vi "Calculate psrr.vi"(8 "error in (no error)":errorcluster, 11 "Time signal(s) in":waveform(dbl)[](array[waveform])) -> (0 "error out":errorcluster, 2 "PSRR":dbl)   [LabVIEW 2021]
uses:
  <vilib>/measure/madcrms.llb/Basic Averaged DC-RMS for N Chan.vi
  <vilib>/measure/NI_MAPro.lvlib
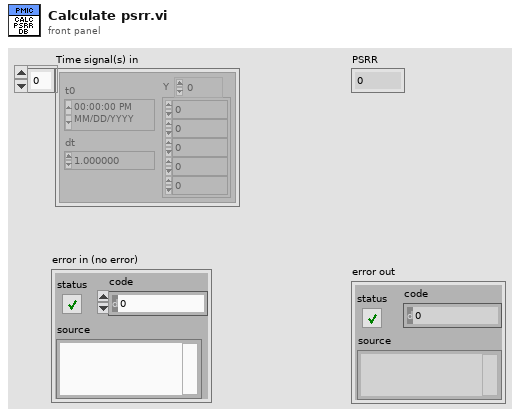
[diagram p1: front panel]
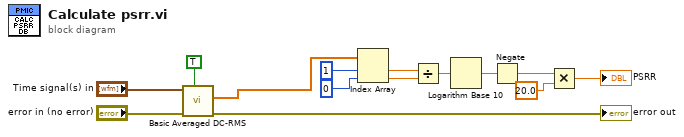
[diagram p0: block diagram]
diagram:
  n1 = call-poly <vilib>:"Basic Averaged DC-RMS.vi"("reset"=TRUE, "error in (no error)"="error in (no error)", "signals in"="Time signal(s) in") -> ("error out"=→"error out":errorcluster, "RMS values"=w13:dbl[])  [unwired: 5 in, 2 out]
  n2 = Index Array(array=w13, index #1=1 ("index"), index #2=0 ("index")) -> (element #1=w9:dbl, element #2=w10:dbl)
  n3 = Divide(x=w9, y=w10) -> (x/y=w8:dbl)
  n4 = Logarithm Base 10(1:w8) -> (0:w7:dbl)
  n5 = Negate(x=w7) -> (-x=w5:dbl)
  n6 = Multiply(x=w5, y=20.0) -> (x*y=→"PSRR":dbl)
